vi "Bitwise NOT (Greyscale with Mask).vi"(8 "error in (no error)":errorcluster, 9 "Mask":T1, 10 "Greyscale Image Destination":T1, 11 "Greyscale Image Source":T1) -> (0 "error out":errorcluster, 3 "Greyscale Image Destination (duplicate)":T1)   [LabVIEW 2020, in "g_ar_toolkit.image.lvlib"]
uses:
  g_ar_toolkit.image.lvlib
  Greyscale Image.ctl
  f9ee80d6-438b-4cfb-91f1-04b98ac80474.vi
  g_ar_toolkit.common/Module Path.vi
  <vilib>/Utility/error.llb/Error Cluster From Error Code.vi
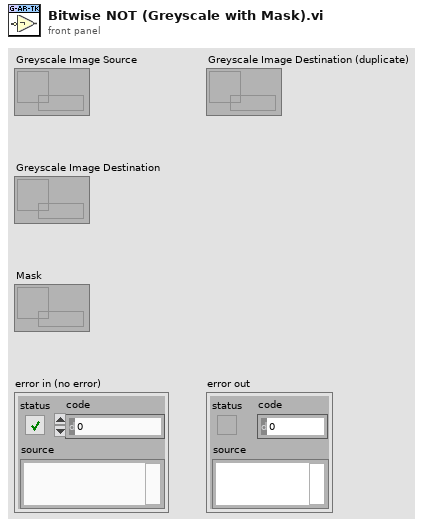
[diagram p1: front panel]
types:
  T1 = typedef "g_ar_toolkit.image.lvlib/Greyscale Image.ctl" = refnum<data-value>
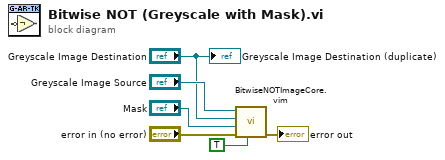
[diagram p0: block diagram]
diagram:
  n1 = call "BitwiseNOTImageCore.vim"("HasMask"=TRUE, "error in (no error)"="error in (no error)", "Mask"="Mask", "Greyscale Image Destination"="Greyscale Image Destination", "Greyscale Image Source"="Greyscale Image Source") -> ("error out"=→"error out":errorcluster)  [unwired: 6 in]
  "Greyscale Image Destination (duplicate)" <- "Greyscale Image Destination"
